vi "DynamicMotionMagicExpoVoltage SetControl.vi"(0 "UseTimesync":bool, 1 "Position":dbl, 2 "kV":dbl, 3 "kA":dbl, 4 "Velocity":dbl, 5 "EnableFOC":bool=TRUE, 6 "FeedForward":dbl, 7 "error in":errorcluster, 8 "Slot":i32, 9 "OverrideBrakeDurNeutral":bool, 10 "LimitForwardMotion":bool, 11 "LimitReverseMotion":bool, 12 "IgnoreHardwareLimits":bool, 13 "IgnoreSoftwareLimits":bool, 18 "Update Frequency (Hz)":dbl=100.0) -> (20 "DeviceReference Out":T1, 27 "error out":errorcluster)   [LabVIEW 2025]
doc: "Requests Motion Magic® Expo to target a final position using an exponential motion profile. This dynamic request allows runtime changes to the profile kV, kA, and (optional) Cruise Velocity. Users can optionally provide a voltage feedforward.\nMotion Magic® Expo produces a motion profile in real-time while attempting to honor the specified Cruise Velocity (optional) and the mechanism kV and kA. Note that unlike the slot gains, the Expo_kV and Expo_kA parameters are always in output units of Volts.\nSetting the Cruise Velocity to 0 will allow the profile to run to the max possible velocity based on Expo_kV. This control mode does not use the Acceleration or Jerk configs.\nTarget position can be changed on-the-fly and Motion Magic® will do its best to adjust the profile. This control mode is voltage-based, so relevant closed-loop gains will use Volts for the numerator."
uses:
  <vilib>/Rock Robotics/WPI/ThirdParty/Phoenix6/DeviceReference.ctl
panel:
  in  "DeviceReference":T1
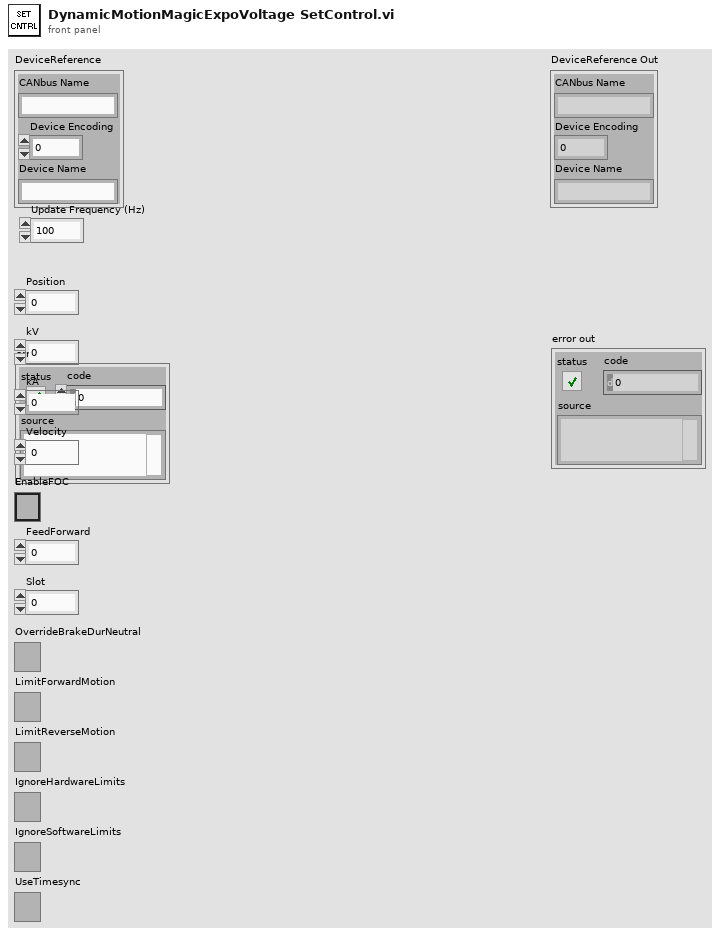
[diagram p1: front panel]
types:
  T1 = typedef "DeviceReference.ctl" = cluster{"CANbus Name":string, "Device Encoding":u32, "Device Name":string}
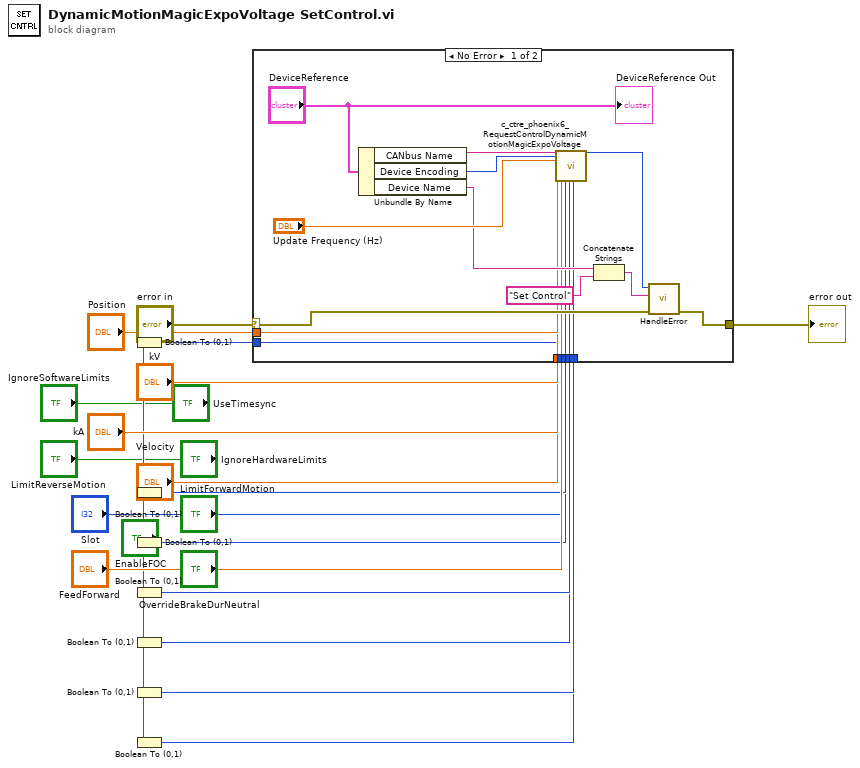
[diagram p0: block diagram]
diagram:
  n1 = Boolean To (0,1)(Boolean="EnableFOC") -> (0, 1=w15:i16)
  n2 = Boolean To (0,1)(Boolean="OverrideBrakeDurNeutral") -> (0, 1=w11:i16)
  n3 = Boolean To (0,1)(Boolean="LimitForwardMotion") -> (0, 1=w9:i16)
  n4 = Boolean To (0,1)(Boolean="LimitReverseMotion") -> (0, 1=w7:i16)
  n5 = Boolean To (0,1)(Boolean="IgnoreHardwareLimits") -> (0, 1=w5:i16)
  n6 = Boolean To (0,1)(Boolean="IgnoreSoftwareLimits") -> (0, 1=w3:i16)
  n7 = Boolean To (0,1)(Boolean="UseTimesync") -> (0, 1=w1:i16)
  n8 = case shown="No Error" "error in" {
    selector: "error in" -> [w40 w46]
    tunnel: [w39 w46] -> w21
    tunnel: "Position" -> [w35 _]
    tunnel: "kV" -> [w34 _]
    tunnel: "kA" -> [w33 _]
    tunnel: "Velocity" -> [w32 _]
    tunnel: w15 -> [w31 _]
    tunnel: "FeedForward" -> [w30 _]
    tunnel: "Slot" -> [w29 _]
    tunnel: w11 -> [w28 _]
    tunnel: w9 -> [w27 _]
    tunnel: w7 -> [w26 _]
    tunnel: w5 -> [w25 _]
    tunnel: w3 -> [w24 _]
    tunnel: w1 -> [w23 _]
    frame No Error {
      n9 = Unbundle By Name("DeviceReference") -> ("CANbus Name"=w44:string, "Device Encoding"=w43:u32, "Device Name"=w38:string)
      n10 = call <vilib>:"c_ctre_phoenix6_RequestControlDynamicMotionMagicExpoVoltage.vi"("String 2"=w44, "Numeric 2"=w43, "Numeric 3"="Update Frequency (Hz)", "Numeric 4"=w35, "Numeric 5"=w34, "Numeric 6"=w33, "Numeric 7"=w32, "Numeric 8"=w31, "Numeric 9"=w30, "Numeric 10"=w29, "Numeric 11"=w28, "Numeric 12"=w27, "Numeric 13"=w26, "Numeric 14"=w25, "Numeric 15"=w24, "Numeric 16"=w23) -> ("Numeric"=w41:i32)  [unwired: 10 in, 1 out]
      n11 = Concatenate Strings(w38, "Set Control" ("origin")) -> (w36:string)
      n12 = call <vilib>:"HandleError.vi"("error in"=w40, "origin"=w36, "Status"=w41) -> ("error out"=w39:errorcluster)  [unwired: 8 in]
      "DeviceReference Out" <- "DeviceReference"
    }
    frame Error {
    }
  }
  "error out" <- w21
